vi "Receive Value Change Event.vi"(8 "error in (no error)":errorcluster, 10 "ValueChangeMsg":refnum<class "ValueChangeMsg.lvclass">, 11 "View Manager In":refnum<class "View Manager.lvclass">=refnum) -> (0 "error out":errorcluster, 3 "View Manager Out":refnum<class "View Manager.lvclass">)   [LabVIEW 2017, in "View Manager.lvlib" / "View Manager.lvclass"]
doc: "<License>\nCopyright © 2017 Composed Systems, LLC | All rights reserved\nwww.composed.io\n\nAuthor: Ethan Stern <ethan.stern@composed.io>\n\nThis software is provided \"AS IS\" WITHOUT WARRANTIES, either express or implied, AND IS FOR EDUCATIONAL PURPOSES ONLY.\n</License>"
uses:
  View Manager.lvclass
  <vilib>/gpm_packages/@cs/mva-viewable/Source/ActorEvents/IEventAggregator Messages/ValueChangeMsg/ValueChangeMsg.lvclass
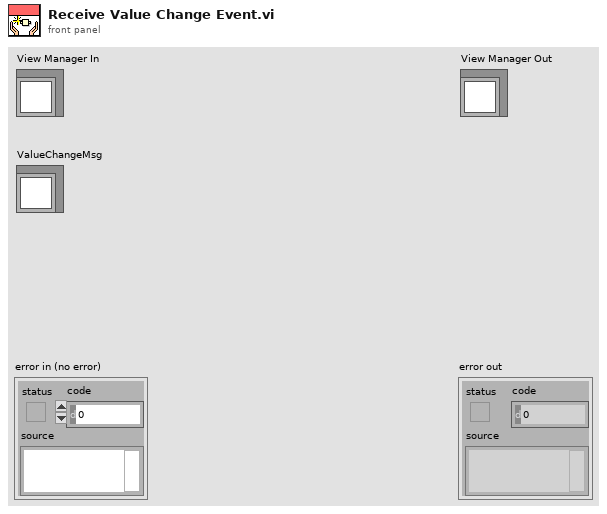
[diagram p1: front panel]
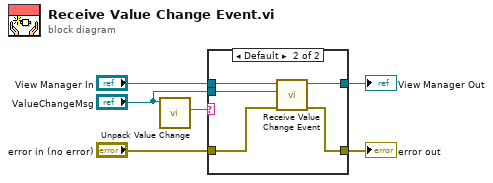
[diagram p0: block diagram]
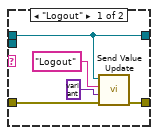
[diagram p2: hidden frame]
diagram:
  n1 = call <vilib>:"Unpack Value Change.vi"("ValueChangeMsg"="ValueChangeMsg") -> ("Control Label"=w1:string)  [unwired: 6 in, 4 out]
  n2 = case shown="Default" w1 {
    tunnel: "View Manager In" -> [w9 w16]
    tunnel: [w9 w15] -> w5
    tunnel: "ValueChangeMsg" -> [_ w14]
    tunnel: "error in (no error)" -> [w7 w13]
    tunnel: [w11 w12] -> w3
    frame "Logout" {
      n3 = call-dynamic "Send Value Update.vi"("error in (no error)"=w7, "Value"=variant, "Datum Name"="Logout", "IViewable in"=w9) -> ("error out"=w11:errorcluster)  [unwired: 7 in]
    }
    frame Default {
      n4 = call-parent "Receive Value Change Event.vi"("error in (no error)"=w13, "ValueChangeMsg"=w14, "IViewable In"=w16) -> ("error out"=w12:errorcluster, "IViewable Out"=w15:refnum<class "View Manager.lvclass">)  [unwired: 7 in]
    }
  }
  "error out" <- w3
  "View Manager Out" <- w5
